vi "Write_coeff.vi"(0 "C\n(Ax^2+Bx+C)":dbl=360.60296, 1 "A\n(Ax^2+Bx+C)":dbl=5.88212e-06, 2 "B\n(Ax^2+Bx+C)":dbl=0.13277, 3 "bck: a\n(ax+b)":dbl=10.39524, 4 "bck: b\n(ax+b)":dbl=465.88005, 5 "address_buffer":u16, 6 "address_flash":u16, 7 "DevDet":i32=1) -> ()   [LabVIEW 2022 SP3]
uses:
  adcDLL_0001.dll
panel:
  out "output array":u8[](array[numeric]) format="%x"
  out "initialized array":u8[](array[numeric])
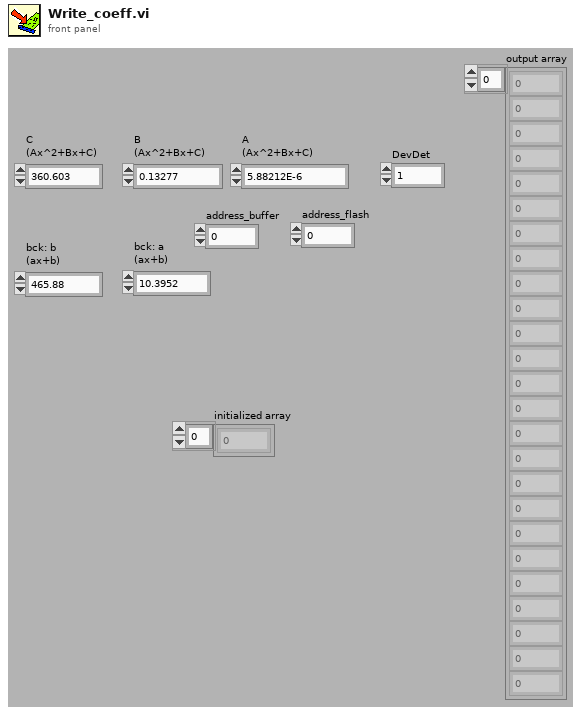
[diagram p1: front panel]
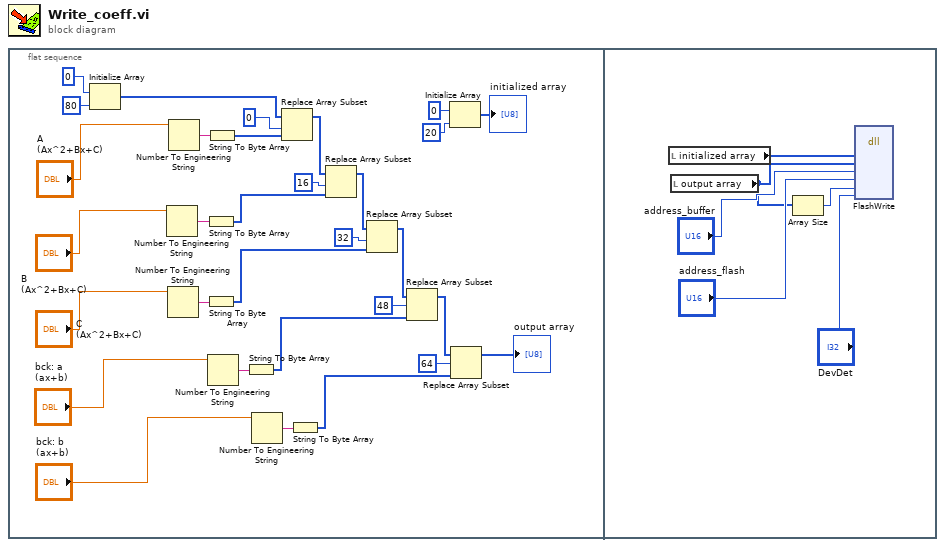
[diagram p0: block diagram]
diagram:
  n1 = flat-sequence {
    frame #0 {
      n2 = Initialize Array(u8 0, 80 ("dimension size")) -> (w20:u8[])
      n3 = Number To Engineering String(4:"B\n(Ax^2+Bx+C)") -> (0:w22:string)  [unwired: 3 in]
      n4 = Number To Engineering String(4:"C\n(Ax^2+Bx+C)") -> (0:w21:string)  [unwired: 3 in]
      n5 = Number To Engineering String(4:"A\n(Ax^2+Bx+C)") -> (0:w23:string)  [unwired: 3 in]
      n6 = String To Byte Array(string=w22) -> (unsigned byte array=w16:u8[])
      n7 = String To Byte Array(string=w21) -> (unsigned byte array=w13:u8[])
      n8 = String To Byte Array(string=w23) -> (unsigned byte array=w19:u8[])
      n9 = Number To Engineering String(4:"bck: a\n(ax+b)") -> (0:w11:string)  [unwired: 3 in]
      n10 = String To Byte Array(string=w11) -> (unsigned byte array=w10:u8[])
      n11 = Number To Engineering String(4:"bck: b\n(ax+b)") -> (0:w7:string)  [unwired: 3 in]
      n12 = Replace Array Subset(array=w20, new element=w19, index=0) -> (w17:u8[])
      n13 = String To Byte Array(string=w7) -> (unsigned byte array=w6:u8[])
      n14 = Replace Array Subset(array=w17, new element=w16, index=16) -> (w14:u8[])
      n15 = Replace Array Subset(array=w14, new element=w13, index=32) -> (w8:u8[])
      n16 = Replace Array Subset(array=w8, new element=w10, index=48) -> (w4:u8[])
      n17 = Initialize Array(u8 0 ("element"), 20 ("dimension size")) -> (→"initialized array":u8[])
      n18 = Replace Array Subset(array=w4, new element=w6, index=64) -> (→"output array":u8[])
    }
    frame #1 {
      n19 = local read "initialized array"() -> (w37:u8[])
      n20 = local read "output array"() -> (w32:u8[])
      n21 = Array Size(array=w32) -> (size(s)=w33:i32)
      n22 = dll-call lib="D:/LabVIEWSuite_64_OS/Spectrometers/ASEQ LR1/adcDLL_0001.dll" fn="FlashWrite"("OutputReport1"=w37, "OutputData1"=w32, "address_buffer"="address_buffer", "address_flash"="address_flash", "length"=w33, "DevDet"="DevDet") -> ()  [unwired: 10 in, 2 out]
    }
  }
